vi "Trace Statistic Analysis Result.vi"(7 "Channel (1)":i32=1, 8 "error in (no error)":errorcluster, 11 "VISA resource name":refnum<visa-resource-name>) -> (0 "error out":errorcluster, 1 "Mean":dbl format="%^.2e", 2 "Standard Deviation":dbl format="%^.2e", 3 "VISA resource name out":refnum<visa-resource-name>, 4 "Peak to Peak":dbl format="%^.2e")   [LabVIEW 2020, in "Agilent ENA Series.lvlib"]
doc: "Reads the number of ports (7 or 9) of the E5091A whose ID is specified in Multiplexer control."
uses:
  <instrlib>/Agilent ENA Series/Agilent ENA Series.lvlib
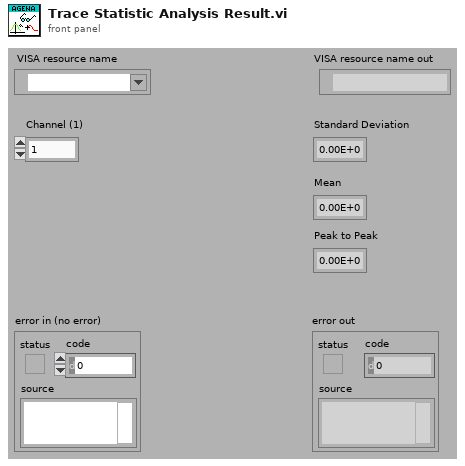
[diagram p1: front panel]
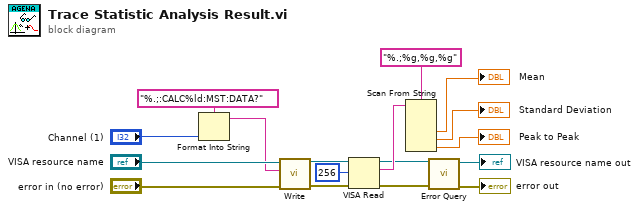
[diagram p0: block diagram]
diagram:
  n1 = Format Into String(format string="%.;:CALC%ld:MST:DATA?", "Channel (1)") -> (resulting string=w14:string)  [unwired: 2 in, 1 out]
  n2 = call <instrlib>:"Write.vi"("error in (no error)"="error in (no error)", "String ()"=w14, "VISA resource name"="VISA resource name") -> ("error out"=w12:errorcluster, "VISA resource name out"=w13:refnum<visa-resource-name>)  [unwired: 6 in, 1 out]
  n3 = VISA Read(VISA resource name=w13, byte count=u32 256, error in (no error)=w12) -> (VISA resource name out=w4:refnum<visa-resource-name>, read buffer=w9:string, error out=w3:errorcluster)  [unwired: 1 out]
  n4 = Scan From String(format string="%.;%g,%g,%g", input string=w9) -> (output 1=→"Mean":dbl, output 2=→"Standard Deviation":dbl, output 3=→"Peak to Peak":dbl)  [unwired: 5 in, 3 out]
  n5 = call <instrlib>:"Error Query.vi"("error in (no error)"=w3, "VISA resource name"=w4) -> ("error out"=→"error out":errorcluster, "VISA resource name out"=→"VISA resource name out":refnum<visa-resource-name>)  [unwired: 6 in, 2 out]
